vi "Write VI Snippet.vi"(8 "error in (no error)":errorcluster, 9 "Image Data":T1, 10 "VI Path (.vi)":path, 11 "VI Snippet (.png)":path) -> (0 "error out":errorcluster)   [LabVIEW 2018, in "Export-Built-ins.lvlib"]
uses:
  Export-Built-ins.lvlib
  <vilib>/picture/picture.llb/imagedata.ctl
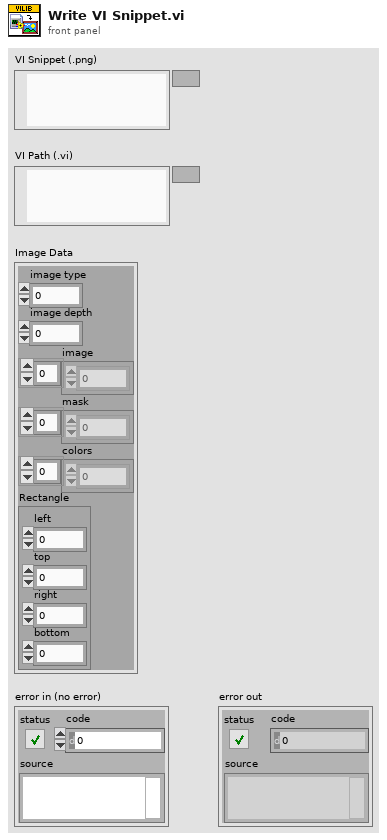
[diagram p1: front panel]
types:
  T1 = typedef "imagedata.ctl" = cluster{"image type":i32, "image depth":i32, "image":u8[], "mask":u8[], "colors":u32[], "Rectangle":cluster{"left":i16, "top":i16, "right":i16, "bottom":i16}}
  T2 = typedef "Export-Built-ins.lvlib/PNG Chunk.ctl" = cluster{"Length":i32, "Type":string, "Data":string, "CRC":u32}
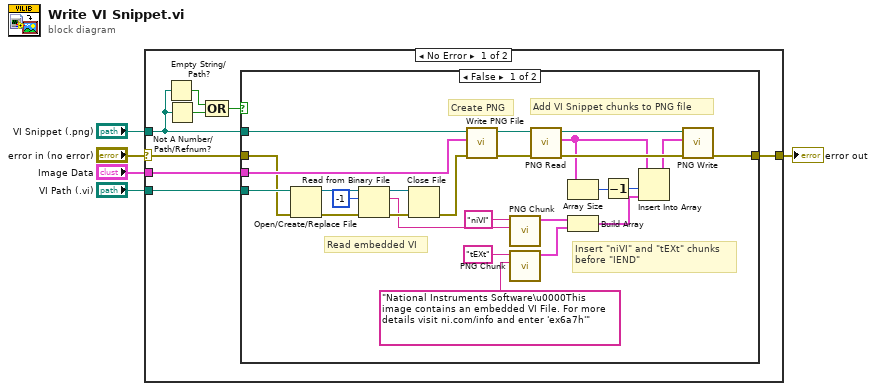
[diagram p0: block diagram]
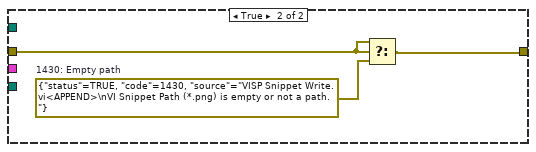
[diagram p2: hidden frame]
diagram:
  n1 = case shown="No Error" "error in (no error)" {
    selector: "error in (no error)" -> [w13 w43]
    tunnel: "VI Snippet (.png)" -> [w10 _]
    tunnel: "Image Data" -> [w12 _]
    tunnel: [w11 w43] -> w4
    tunnel: "VI Path (.vi)" -> [w9 _]
    frame No Error {
      n2 = Empty String/Path?(string/path=w10) -> (empty?=w7:bool)
      n3 = Not A Number/Path/Refnum?(number/path/refnum=w10) -> (NaN/Path/Refnum?=w8:bool)
      n4 = Compound Arithmetic op=OR(w7, w8) -> (w6:bool)
      n5 = case shown="False" w6 {
        tunnel: w13 -> [w16 w42]
        tunnel: w10 -> [w39 _]
        tunnel: w12 -> [w38 _]
        tunnel: [w27 w41] -> w11
        tunnel: w9 -> [w19 _]
        frame False {
          # "Read embedded VI"
          # "Create PNG"
          # "Add VI Snippet chunks to PNG file"
          # "Insert \"niVI\" and \"tEXt\" chunks\nbefore \"IEND\""
          n6 = Open/Create/Replace File(file path (use dialog)=w19, error in=w16) -> (refnum out=w18:refnum<file>, error out=w17:errorcluster)  [unwired: 4 in, 1 out]
          n7 = Read from Binary File(8:w17, 10:-1 ("count (1)"), 11:w18) -> (0:w25:errorcluster, 2:w23:string, 3:w24:refnum<file>)  [unwired: 3 in, 1 out]
          n8 = Close File(refnum=w24, error in=w25) -> (error out=w15:errorcluster)  [unwired: 1 out]
          n9 = call <vilib>:"Write PNG File.vi"("error in (no error)"=w15, "image data"=w38, "path to PNG file"=w39) -> ("error out"=w14:errorcluster, "path"=w22:path)  [unwired: 7 in]
          n10 = call "PNG Chunk.vi"("Data"=w23, "Type"="niVI") -> ("PNG Chunk"=w30:T2)  [unwired: 9 in]
          n11 = call "PNG Chunk.vi"("Data"="National Instruments Software\u0000This image contains an embedded VI File. For more details visit ni.com/info and enter 'ex6a7h'", "Type"="tEXt") -> ("PNG Chunk"=w29:T2)  [unwired: 9 in]
          n12 = call "PNG Read.vi"("error in (no error)"=w14, "Image Path (*.png)"=w22) -> ("error out"=w37:errorcluster, "Chunks"=w21:T2[], "dup Image Path"=w20:path)  [unwired: 7 in]
          n13 = Array Size(array=w21) -> (size(s)=w35:i32)
          n14 = Build Array(w30, w29) -> (w28:T2[])
          n15 = Decrement(x=w35) -> (x-1=w34:i32)
          n16 = Insert Into Array(array=w21, index=w34, new element=w28) -> (w36:T2[])
          n17 = call "PNG Write.vi"("error in (no error)"=w37, "Chunks"=w36, "Image Path (*.png)"=w20) -> ("error out"=w27:errorcluster)  [unwired: 7 in, 1 out]
        }
        frame True {
          w40 = errorcluster {"status"=TRUE, "code"=1430, "source"="VISP Snippet Write.vi<APPEND>\nVI Snippet Path (*.png) is empty or not a path."}  # 1430: Empty path
          n18 = Select(t=w42, s=w42, f=w40) -> (s? t:f=w41:errorcluster)
        }
      }
    }
    frame Error {
    }
  }
  "error out" <- w4
